vi "Ok to proceed check.vi"() -> (0 "Error":errorcluster)   [LabVIEW 2014]
uses:
  Laser enum.ctl
  Commands.ctl
  Coherent global.vi
panel:
  # "PN 06/11/2014"
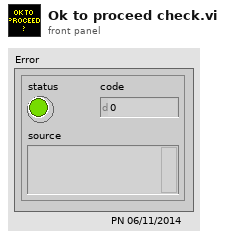
[diagram p1: front panel]
types:
  T1 = typedef "Commands.ctl" = u8
  T2 = typedef "Laser enum.ctl" = u8
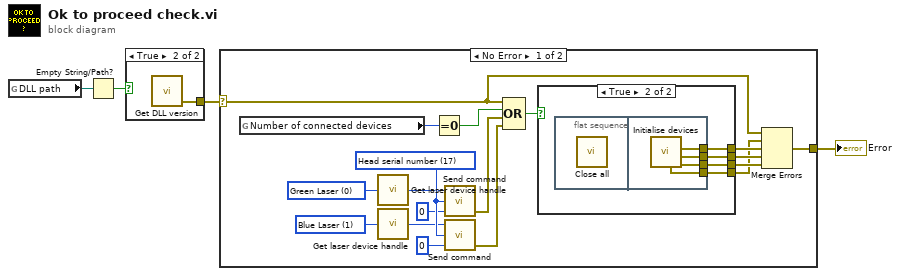
[diagram p0: block diagram]
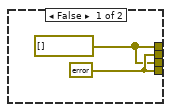
[diagram p2: hidden frame]
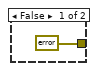
[diagram p4: hidden frame]
diagram:
  n1 = global read "Coherent global.vi" "DLL path"() -> (w3:path)
  n2 = Empty String/Path?(string/path=w3) -> (empty?=w2:bool)
  n3 = case shown="True" w2 {
    tunnel: [errorcluster {"status"=FALSE, "code"=0, "source"=""} ("Error") w6] -> w1
    frame False {
    }
    frame True {
      n4 = call "Get DLL version.vi"() -> ("Error"=w6:errorcluster)  [unwired: 2 out]
    }
  }
  n5 = case shown="No Error" w1 {
    selector: w1 -> [w11 w35]
    tunnel: [w12 w35] -> w4
    frame No Error {
      w21 = T1 17 items=["Measured main TEC temperature"=0, "Measured SHG heater temperature"=1, "Measured BRF heater temperature"=2, "Main TEC temperature command"=3, "SHG heater temperature command"=4, "BRF heater temperature command"=5, "Main TEC drive"=6, "SHG heater drive"=7, "BRF heater drive"=8, "Output power from photodiode"=9, "Output power setpoint (Get)"=10, "Output power setpoint (Set)"=11, "Start-up power setting (Get)"=12, "Start-up power setting (Set)"=13, "Measured LDD current"=14, "Maximum LDD current limit"=15, "16-bit fault code"=16, "Head serial number"=17, "Head board rev"=18, "Head type"=19, "LDD enable state"=20, "Key switch command (Get)"=24, "Key switch command (Set)"=25, "Key switch actual"=26, "Interlock status"=27, "Head hours"=28, "Photo or current mode command (Get)"=29, "Photo or current mode command (Set)"=30, "Photo or current mode actual"=31, "Analog input enable command (Get)"=32, "Analog input enable command (Set)"=33, "Analog input actual"=34, "Power supply glue input"=36, "Power supply glue output"=37] ("Command")
      w8 = T2 1 items=["Green Laser", "Blue Laser"] ("Selected laser")
      w10 = T2 0 items=["Green Laser", "Blue Laser"] ("Selected laser")
      n6 = global read "Coherent global.vi" "Number of connected devices"() -> (w24:u32)
      n7 = call "Get laser device handle.vi"("Selected laser"=w10) -> ("Device handle"=w9:u32)
      n8 = call "Get laser device handle.vi"("Selected laser"=w8) -> ("Device handle"=w7:u32)
      n9 = Equal To 0?(x=w24) -> (x = 0?=w23:bool)
      n10 = call "Send command.vi"("Value"=u16 0, "Command"=w21, "Device handle"=w9) -> ("Error"=w18:errorcluster)  [unwired: 2 out]
      n11 = call "Send command.vi"("Value"=u16 0, "Command"=w21, "Device handle"=w7) -> ("Error"=w17:errorcluster)  [unwired: 2 out]
      n12 = Compound Arithmetic op=OR(w11, w23, w18, w17) -> (w22:bool)
      n13 = case shown="True" w22 {
        tunnel: [w25 w30] -> w16
        tunnel: [w26 w29] -> w15
        tunnel: [w25 w28] -> w14
        tunnel: [w26 w27] -> w13
        frame False {
          w26 = errorcluster {"status"=FALSE, "code"=0, "source"=""} ("Device detection error")
          w25 = errorcluster[] [] ("Device initialisation errors")
        }
        frame True {
          n14 = flat-sequence {
            tunnel: [w34] -> w30
            tunnel: [w33] -> w29
            tunnel: [w32] -> w28
            tunnel: [w31] -> w27
            frame #0 {
              n15 = call "Close all.vi"() -> ()  [unwired: 1 out]
            }
            frame #1 {
              n16 = call "Initialise devices.vi"() -> ("Laser comms. error"=w34:errorcluster[], "Get lasers serial num. error"=w31:errorcluster, "Device detection error"=w33:errorcluster, "Device initialisation errors"=w32:errorcluster[])  [unwired: 5 in, 2 out]
            }
          }
        }
      }
      n17 = Merge Errors(w11, w13, w16, w15, w14) -> (w12:errorcluster)
    }
    frame Error {
    }
  }
  "Error" <- w4
